vi "ReadRate.vi"   [LabVIEW 2016]
uses:
  Program Files/National Instruments/LabVIEW 2019/user.lib/Nanonis Prog Interface V5/Nanonis Prog Interface.lvlib
panel:
  # "Oversampling: Probably has no effect, only affects SNR/aliasing/stuff like that"
  # "TCP Read Rate: probably the one I want"
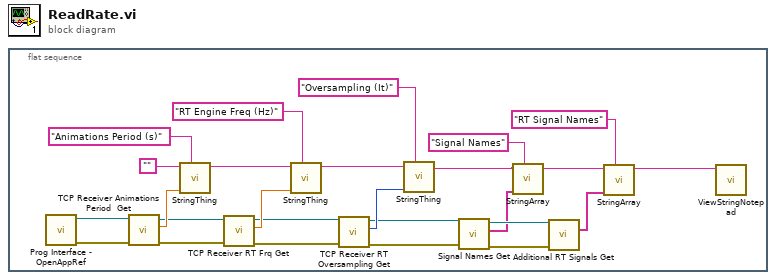
[diagram p0: block diagram]
diagram:
  n1 = flat-sequence {
    frame #0 {
      n2 = call <userlib>:"Prog Interface - OpenAppRef.vi"() -> ("Error out"=w26:errorcluster, "Application reference"=w18:refnum<vi>)  [unwired: 6 in]
      n3 = call <userlib>:"TCP Receiver Animations Period  Get.vi"("Error in (no error)"=w26, "Application ref in"=w18) -> ("Error out"=w25:errorcluster, "Animations Period (s)"=w24:sgl, "Application ref out"=w19:refnum<vi>)  [unwired: 7 in]
      n4 = call "StringThing.vi"("Signal Name"="Animations Period (s)", "Input"=w24, "Carry"="") -> ("Output"=w21:string)  [unwired: 8 in]
      n5 = call <userlib>:"TCP Receiver RT Frq Get.vi"("Error in (no error)"=w25, "Application ref in"=w19) -> ("Error out"=w16:errorcluster, "RT Engine Frq (Hz)"=w20:sgl, "Application ref out"=w17:refnum<vi>)  [unwired: 7 in]
      n6 = call "StringThing.vi"("Signal Name"="RT Engine Freq (Hz)", "Input"=w20, "Carry"=w21) -> ("Output"=w14:string)  [unwired: 8 in]
      n7 = call <userlib>:"TCP Receiver RT Oversampling Get.vi"("Error in (no error)"=w16, "Application ref in"=w17) -> ("Error out"=w11:errorcluster, "Oversampling"=w13:i32, "Application ref out"=w12:refnum<vi>)  [unwired: 7 in]
      n8 = call "StringThing.vi"("Signal Name"="Oversampling (It)", "Input"=w13, "Carry"=w14) -> ("Output"=w8:string)  [unwired: 8 in]
      n9 = call <userlib>:"Signal Names Get.vi"("error in (no error)"=w11, "Application ref in"=w12) -> ("error out"=w9:errorcluster, "Signals Names"=w7:string[], "Application ref out"=w10:refnum<vi>)  [unwired: 5 in]
      n10 = call "StringArray.vi"("Array Name"="Signal Names", "Input"=w7, "Carry"=w8) -> ("Output"=w4:string)  [unwired: 8 in]
      n11 = call <userlib>:"Additional RT Signals Get.vi"("Application ref in"=w10, "error in (no error)"=w9) -> ("Additional RT Signals Names"=w5:string[])  [unwired: 9 in, 4 out]
      n12 = call "StringArray.vi"("Array Name"="RT Signal Names", "Input"=w5, "Carry"=w4) -> ("Output"=w1:string)  [unwired: 8 in]
      n13 = call "ViewStringNotepad.vi"("Input"=w1) -> ()  [unwired: 11 in]
    }
  }
